vi "FUG_PowerSupply.constructor.vi"(0 "name":string, 2 "data in":string, 5 "error in(no error)":errorcluster) -> (14 "i ref out":refnum<vi>, 16 "data out":string, 19 "error out":errorcluster)   [LabVIEW 2014, in "FUG_PowerSupply.lvlib"]
doc: "This is the constructor of a class.\n\nLicense Agreement for this software:\n\nCopyright (C)\nGesellschaft für Schwerionenforschung, GSI\nPlanckstr. 1\n64291 Darmstadt\nGermany\n\nContact: D.Beck@gsi.de \n\nThis program is free software; you can redistribute it and/or modify it under the terms of the \nGNU General Public License as published by the Free Software Foundation; either version 2 of \nthe license, or (at your option) any later version.\n\nThis program is distributed in the hope that it will be useful, but WITHOUT ANY WARRANTY; \nwithout even the implied warranty of MERCHANTABILITY or FITNESS FOR A PARTICULAR PURPOSE. See the GNU General License for more details (http://www.gnu.org).\n\nGesellschaft für Schwerionenforschung, GSI\nPlanckstr. 1, 64291 Darmstadt, Germany\nFor all questions and ideas contact: M.Richter@gsi.de, H.Brand@gsi.de or D.Beck@gsi.de.\nLast update: 16-JUN-2004"
uses:
  FUG_PowerSupply.lvlib
  CSCore/CSApplicationBaseClasses/DeviceBase/DeviceBase.myEventNames.ctl
  CSCore/CSApplicationBaseClasses/PSChannelBase/PSChannelBase.myEventNames.ctl
  CSlibraries/UtilityLib/UtilityLib.valueStatus.ctl
  CSCore/CSSystem/CSSystemLib/CSSystemLib.lvlib
  CSCore/CSApplicationBaseClasses/PSChannelBase/PSChannelBase.lvlib
  CSCore/CSApplicationBaseClasses/DeviceBase/DeviceBase.lvlib
  CSlibraries/UtilityLib/UtilityLib.lvlib
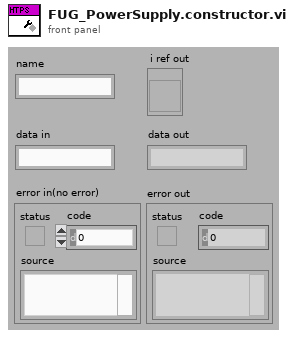
[diagram p1: front panel]
types:
  T1 = typedef "UtilityLib.lvlib/UtilityLib.valueStatus.ctl" = enum16{"no info available", "stand by/off", "on", "warning", "alarm/malfunction", "not implemented", "user action required", "important information", "system default", "control default", "indicator default", "button default"}
  T2 = enum16{"SetAttribute", "GetAttribute", "CreateAttribute", "DestroyAttribute", "DestroyAllAtributes"}
  T3 = typedef "PSChannelBase.lvlib/PSChannelBase.myEventNames.ctl" = enum16{"lvmsg://EmergencyOff", "lvmsg://SetOnOff", "lvmsg://GetOnOff", "lvmsg://SetVoltage", "lvmsg://GetVoltage", "lvmsg://SetCurrent", "lvmsg://GetCurrent", "lvmsg://SetTripCurrent", "lvmsg://GetTripCurrent", "lvmsg://SetRampUpSpeed", "lvmsg://GetRampUpSpeed", "lvmsg://SetRampDownSpeed", "lvmsg://GetRampDownSpeed", "lvmsg://SetChannelOnOff", "lvmsg://GetChannelOnOff", "lvmsg://SetChannelVoltage", "lvmsg://GetChannelVoltage", "lvmsg://SetChannelCurrent", "lvmsg://GetChannelCurrent", "lvmsg://SetChannelTripCurrent", "lvmsg://GetChannelTripCurrent", "lvmsg://SetChannelRampUpSpeed", "lvmsg://GetChannelRampUpSpeed", "lvmsg://SetChannelRampDownSpeed", "lvmsg://GetChannelRampDownSpeed"}
  T4 = typedef "DeviceBase.lvlib/DeviceBase.myEventNames.ctl" = enum16{"lvmsg://Initialize", "lvmsg://Close", "lvmsg://Configure", "lvmsg://Reset", "lvmsg://IDQuery"}
  T5 = typedef "FUG_PowerSupply.lvlib/FUG_PowerSupply.i attribute.ctl" = cluster{"Type":string, "Elektrode Name":string, "CALC_FACTOR_SET_VOLTAGE":dbl, "CALC_FACTOR_GET_VOLTAGE":dbl, "CALC_FACTOR_GET_CURRENT":dbl, "CALC_FACTOR_SET_CURRENT ":dbl, "REG_VALUE":dbl, "Sign":bool, "setVoltID":i32, "setCurrentID":i32, "setPowerOnID":i32, "MaxVoltage":dbl}
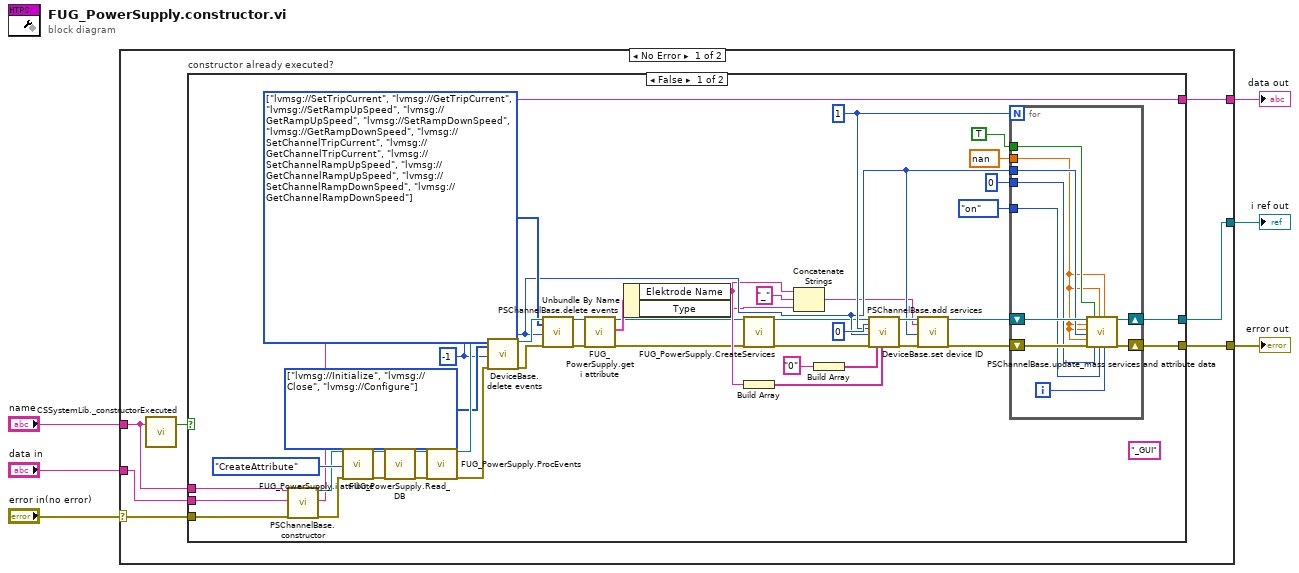
[diagram p0: block diagram]
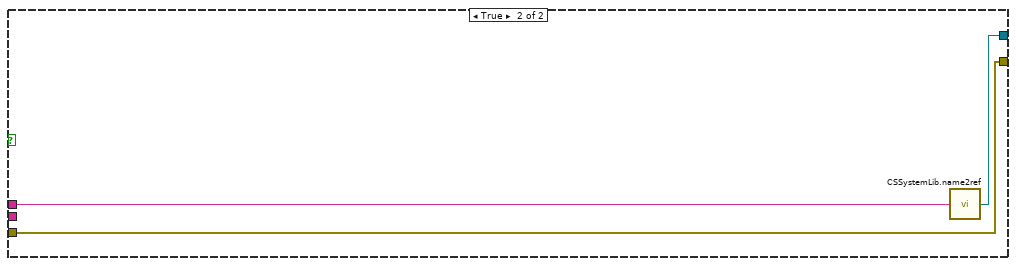
[diagram p2: hidden frame]
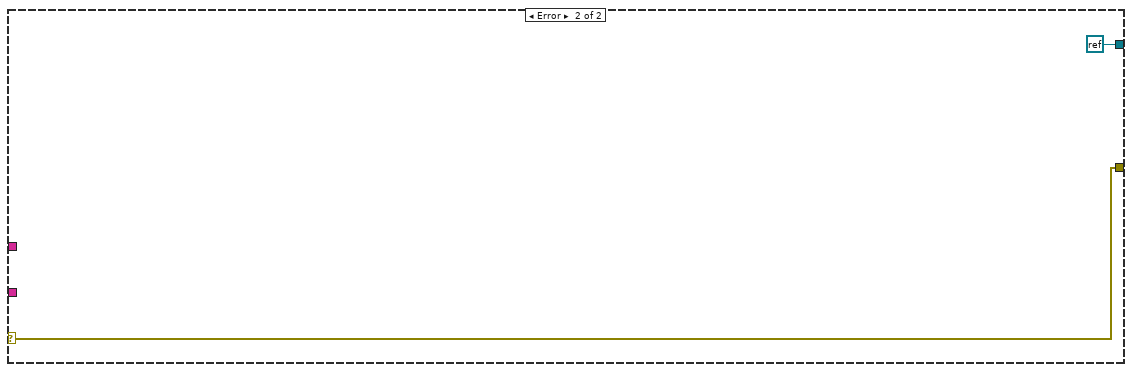
[diagram p3: hidden frame]
diagram:
  n1 = case shown="No Error" "error in(no error)" {
    selector: "error in(no error)" -> [w11 w71]
    tunnel: "name" -> [w10 _]
    tunnel: [w13 refnum<k0> refnum] -> w5
    tunnel: [w12 w71] -> w4
    tunnel: "data in" -> [w8 _]
    tunnel: [w7 _] -> w1
    frame No Error {
      n2 = call "CSSystemLib._constructorExecuted.vi"("name"=w10) -> ("constructor executed?"=w9:bool)  [unwired: 18 in]
      n3 = case "constructor already executed?" shown="False" w9 {
        tunnel: [w33 w69] -> w13
        tunnel: [w34 w68] -> w12
        tunnel: w11 -> [w57 w68]
        tunnel: w10 -> [w16 w70]
        tunnel: w8 -> [w56 _]
        tunnel: [w50 _] -> w7
        frame False {
          (unwired) "_GUI" ("string")
          w42 = T3[] [enum."lvmsg://SetTripCurrent", enum."lvmsg://GetTripCurrent", enum."lvmsg://SetRampUpSpeed", enum."lvmsg://GetRampUpSpeed", enum."lvmsg://SetRampDownSpeed", enum."lvmsg://GetRampDownSpeed", enum."lvmsg://SetChannelTripCurrent", enum."lvmsg://GetChannelTripCurrent", enum."lvmsg://SetChannelRampUpSpeed", enum."lvmsg://GetChannelRampUpSpeed", enum."lvmsg://SetChannelRampDownSpeed", enum."lvmsg://GetChannelRampDownSpeed"] items=["lvmsg://EmergencyOff", "lvmsg://SetOnOff", "lvmsg://GetOnOff", "lvmsg://SetVoltage", "lvmsg://GetVoltage", "lvmsg://SetCurrent", "lvmsg://GetCurrent", "lvmsg://SetTripCurrent", "lvmsg://GetTripCurrent", "lvmsg://SetRampUpSpeed", "lvmsg://GetRampUpSpeed", "lvmsg://SetRampDownSpeed", "lvmsg://GetRampDownSpeed", "lvmsg://SetChannelOnOff", "lvmsg://GetChannelOnOff", "lvmsg://SetChannelVoltage", "lvmsg://GetChannelVoltage", "lvmsg://SetChannelCurrent", "lvmsg://GetChannelCurrent", "lvmsg://SetChannelTripCurrent", "lvmsg://GetChannelTripCurrent", "lvmsg://SetChannelRampUpSpeed", "lvmsg://GetChannelRampUpSpeed", "lvmsg://SetChannelRampDownSpeed", "lvmsg://GetChannelRampDownSpeed"] ("events")
          w45 = T4[] [enum."lvmsg://Initialize", enum."lvmsg://Close", enum."lvmsg://Configure"] items=["lvmsg://Initialize", "lvmsg://Close", "lvmsg://Configure", "lvmsg://Reset", "lvmsg://IDQuery"] ("events")
          w29 = 1 ("nofChannels")
          w25 = -1 ("ms timeout (10000)")
          n4 = call "PSChannelBase.constructor.vi"("name"=w16, "data in"=w56, "error in (no error)"=w57) -> ("i ref out"=w51:refnum<vi>, "data out"=w50:string, "error out"=w52:errorcluster)  [unwired: 14 in]
          n5 = call "FUG_PowerSupply.i attribute.vi"("VI Refnum"=w51, "Action"=T2."CreateAttribute", "error in (no error)"=w52) -> ("VI Refnum out"=w54:refnum<vi>, "error out"=w53:errorcluster)  [unwired: 14 in, 1 out]
          n6 = call "FUG_PowerSupply.Read_DB.vi"("i ref in"=w54, "error in (no error)"=w53) -> ("i ref out"=w49:refnum<vi>, "error out (no error)"=w48:errorcluster)  [unwired: 16 in]
          n7 = call "FUG_PowerSupply.ProcEvents.vi"("i ref in"=w49, "error in"=w48) -> ("i ref out"=w47:refnum<vi>, "error out"=w46:errorcluster)  [unwired: 16 in]
          n8 = call "DeviceBase.delete events.vi"("i ref in"=w47, "events"=w45, "ms timeout (10000)"=w25, "error in (no error)"=w46) -> ("i ref out"=w44:refnum<vi>, "error out"=w43:errorcluster)  [unwired: 13 in, 1 out]
          n9 = call "PSChannelBase.delete events.vi"("i ref in"=w44, "events"=w42, "ms timeout (10000)"=w25, "error in (no error)"=w43) -> ("i ref out"=w39:refnum<vi>, "error out"=w40:errorcluster)  [unwired: 13 in, 1 out]
          n10 = call "FUG_PowerSupply.get i attribute.vi"("i ref in"=w39, "error in (no error)"=w40) -> ("i ref out"=w14:refnum<vi>, "i attribute"=w38:T5, "error out"=w15:errorcluster)  [unwired: 15 in]
          n11 = Unbundle By Name(w38) -> ("Elektrode Name"=w24:string, "Type"=w18:string)
          n12 = call "FUG_PowerSupply.CreateServices.vi"("i ref in"=w14, "error in(no error)"=w15) -> ("i ref out"=w19:refnum<vi>, "error out"=w20:errorcluster)  [unwired: 16 in]
          n13 = Build Array(w24) -> (w35:string[])
          n14 = Concatenate Strings(w24, "_" ("string"), w18) -> (w22:string)
          n15 = Build Array("0") -> (w36:string[])
          n16 = call "PSChannelBase.add services.vi"("i ref in"=w19, "defaultChannelIndex"=0, "nofChannels"=w29, "ms timeout (10000)"=w25, "error in (no error)"=w20, "physicalNames"=w36, "logicalNames"=w35) -> ("i ref out"=w28:refnum<vi>, "error out"=w26:errorcluster)  [unwired: 10 in, 1 out]
          n17 = call "DeviceBase.set device ID.vi"("i ref in"=w28, "deviceID"=w22, "ms timeout (10000)"=w25, "error in (no error)"=w26) -> ("i ref out"=w27:refnum<vi>, "error out"=w21:errorcluster)  [unwired: 13 in, 1 out]
          n18 = for {
            N: w29 -> [_]
            shift-right: [w65] -> w34
            shift-left: w21 -> [w66]
            shift-right: [w63] -> w33
            shift-left: w27 -> [w64]
            tunnel: UtilityLib.valueStatus."on" ("valueStatus") -> [w62]
            tunnel: nan -> [w59]
            tunnel: w25 -> [w61]
            tunnel: TRUE -> [w60]
            tunnel: 0 -> [w58]
            i -> [w67]
            n19 = call "PSChannelBase.update_mass services and attribute data.vi"("i ref in"=w64, "tripCurrent"=w59, "rampUpSpeed"=w59, "ms timeout (10000)"=w61, "rampDownSpeed"=w59, "error in (no error)"=w66, "onOff"=w60, "status"=w58, "voltage"=w59, "valueStatus"=w62, "current"=w59, "channelNumber"=w67) -> ("i ref out"=w63:refnum<vi>, "error out"=w65:errorcluster)  [unwired: 5 in, 1 out]
          }
        }
        frame True {
          n20 = call "CSSystemLib.name2ref.vi"("name"=w70) -> ("obj refnum"=w69:refnum<vi>)
        }
      }
    }
    frame Error {
    }
  }
  "i ref out" <- w5
  "error out" <- w4
  "data out" <- w1
